vi "Parse Field.vi"(8 "error in (no error)":errorcluster, 10 "Text":string, 11 "ProtoParser in":refnum<class "ProtoParser.lvclass">) -> (0 "error out":errorcluster, 2 "Field":T1={"Name"="", "Number"=0, "Optional"=FALSE, "Repeated"=FALSE, "Type"={"Type"=enum."double", "Subtype"=""}, "Key Type"={"Type"=enum."double", "Subtype"=""}, "Value Type"={"Type"=enum."double", "Subtype"=""}}, 3 "ProtoParser out":refnum<class "ProtoParser.lvclass">)   [LabVIEW 2020, in "LV-Protoc.lvlib" / "ProtoParser.lvclass"]
uses:
  ProtoParser.lvclass
  LV-Proto/Field.ctl
  LV-Proto/Type.ctl
  LV-Proto/Proto Type.ctl
  LV-Proto/LV-Proto.lvlib
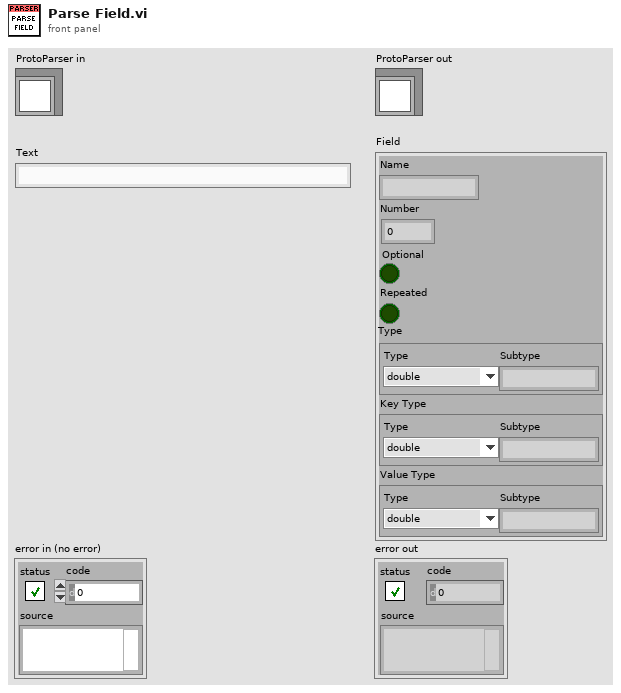
[diagram p1: front panel]
types:
  T1 = typedef "LV-Proto.lvlib/Field.ctl" = cluster{"Name":string, "Number":u32, "Optional":bool, "Repeated":bool, "Type":T2, "Key Type":T2, "Value Type":T2}
  T2 = typedef "LV-Proto.lvlib/Type.ctl" = cluster{"Type":T3, "Subtype":string}
  T3 = typedef "LV-Proto.lvlib/Proto Type.ctl" = enum16{"UNKNOWN", "double", "float", "int32", "int64", "uint32", "uint64", "sint32", "sint64", "fixed32", "fixed64", "sfixed32", "sfixed64", "bool", "string", "bytes", "enum", "map", "message"}
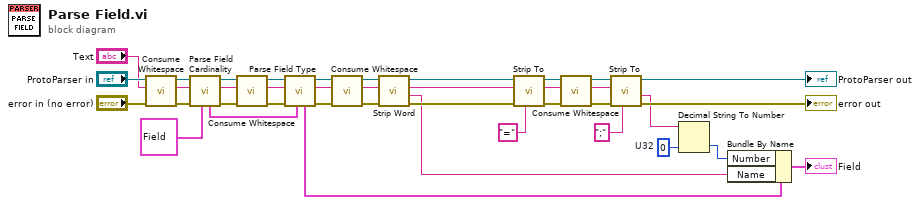
[diagram p0: block diagram]
diagram:
  w23 = u32 0  # U32
  n1 = call "Consume Whitespace.vi"("error in (no error)"="error in (no error)", "String"="Text", "ProtoParser in"="ProtoParser in") -> ("error out"=w16:errorcluster, "Remaining"=w9:string, "ProtoParser out"=w10:refnum<class "ProtoParser.lvclass">)  [unwired: 6 in]
  n2 = call "Parse Field Cardinality.vi"("Field in"=T1 {"Name"="", "Number"=0, "Optional"=FALSE, "Repeated"=FALSE, "Type"={"Type"=enum."double", "Subtype"=""}, "Key Type"={"Type"=enum."double", "Subtype"=""}, "Value Type"={"Type"=enum."double", "Subtype"=""}} ("Field"), "error in (no error)"=w16, "Text"=w9, "ProtoParser in"=w10) -> ("error out"=w4:errorcluster, "Remaining"=w5:string, "ProtoParser out"=w6:refnum<class "ProtoParser.lvclass">, "Field"=w8:T1)  [unwired: 4 in]
  n3 = call "Consume Whitespace.vi"("error in (no error)"=w4, "String"=w5, "ProtoParser in"=w6) -> ("error out"=w3:errorcluster, "Remaining"=w2:string, "ProtoParser out"=w1:refnum<class "ProtoParser.lvclass">)  [unwired: 6 in]
  n4 = call "Parse Field Type.vi"("Field in"=w8, "error in (no error)"=w3, "Text"=w2, "ProtoParser in"=w1) -> ("error out"=w15:errorcluster, "Remaining"=w21:string, "ProtoParser out"=w22:refnum<class "ProtoParser.lvclass">, "Field"=w19:T1)  [unwired: 4 in]
  n5 = call "Consume Whitespace.vi"("error in (no error)"=w15, "String"=w21, "ProtoParser in"=w22) -> ("error out"=w14:errorcluster, "Remaining"=w26:string, "ProtoParser out"=w27:refnum<class "ProtoParser.lvclass">)  [unwired: 6 in]
  n6 = call "Strip Word.vi"("error in (no error)"=w14, "String"=w26, "ProtoParser in"=w27) -> ("error out"=w38:errorcluster, "Word"=w20:string, "Remaining"=w24:string, "ProtoParser out"=w25:refnum<class "ProtoParser.lvclass">)  [unwired: 5 in]
  n7 = call "Strip To.vi"("End"="=", "error in (no error)"=w38, "String"=w24, "ProtoParser in"=w25) -> ("error out"=w13:errorcluster, "Remaining"=w33:string, "ProtoParser out"=w34:refnum<class "ProtoParser.lvclass">)  [unwired: 4 in, 1 out]
  n8 = call "Consume Whitespace.vi"("error in (no error)"=w13, "String"=w33, "ProtoParser in"=w34) -> ("error out"=w12:errorcluster, "Remaining"=w31:string, "ProtoParser out"=w32:refnum<class "ProtoParser.lvclass">)  [unwired: 6 in]
  n9 = call "Strip To.vi"("End"=";", "error in (no error)"=w12, "String"=w31, "ProtoParser in"=w32) -> ("error out"=→"error out":errorcluster, "Portion"=w29:string, "ProtoParser out"=→"ProtoParser out":refnum<class "ProtoParser.lvclass">)  [unwired: 4 in, 1 out]
  n10 = Decimal String To Number(string=w29, default (0L)=w23) -> (number=w18:u32)  [unwired: 1 in, 1 out]
  n11 = Bundle By Name(cluster=w19, "Number"=w18, "Name"=w20) -> (→"Field":T1)
